vi "PROCEDURA TORSIOMETRO.vi"(6 "Text.Text":string="Prova QH: ", 7 "Tipo motore pompa":enum16{"Monofase", "Trifase"}(ring), 9 "Manuale F\\auto T":bool=TRUE, 10 "Status":refnum<vi>, 11 "input cluster":T1={"Scelta wattmetro"={"Wattmetro"=enum."No Selection"}, "SET RPM"=0.0, "SET TEMP"=0.0, "Array banchi"=[{"Nome"="Elettropompa", "Tors. scala1"=0, "Tors. scala2"=0, "rpm"=0, "TAMB"=0, "Indici Temperature"=[0, 1], "Indice freno"=1, "alimentatore trifase"=0, "alimentatore monofase"=0, "alimentatore dc arm"=0, "alimentatore dc ecc"=0, "alimentatore dc mp"=0}, {"Nome"="Sommersa", "Tors. scala1"=0, "Tors. scala2"=0, "rpm"=0, "TAMB"=1, "Indici Temperature"=[0, 1], "Indice freno"=0, "alimentatore trifase"=0, "alimentatore monofase"=0, "alimentatore dc arm"=0, "alimentatore dc ecc"=0, "alimentatore dc mp"=0}], "Array valvole linee avvio/fermata"=[], "banco selezionato"=0, "Nomi valvole prop sistema"=[], "canale-- sensore"=[], "Attriti B1"=[], "Attriti B2"=[], "Collegamento elettrico"={"ALIMENTAZIONE ELETTRICA"=enum."AC MONOFASE", "ID"=0, "#rami freddo\\eq term resmeter"=0, "#rami riscaldamento resmeter"=0, "#rami freddo\\eq term resistomat"=0, "#rami riscaldamento resistomat"=0, "CALCOLI"=enum."AC TRIFASE"}, "lingua"=0, "Costanti collaudo"={"P [bar]"=0.0, "T amb. [°C]"=0.0, "Umidità [%]"=0.0, "T acqua [°C] 2"=0.0}, "OPZIONI MISURE RES"={"MISURA A FREDDO"=enum."RESISTOMAT", "MISURA EQ. TERMICO"=enum."RESISTOMAT", "MISURA DT PROVA IN CORSO"=enum."RESISTOMAT - CON FERMATE", "MISURE PRIMA E DOPO"=enum."RESISTOMAT", "STRUMENTI PRESENTI"=enum."NESSUNO"}, "Dati targa motore"={"Vnom"=0.0, "Fnom"=0.0, "Inom"=0.0, "Cnom"=0.0, "Npoli"=0.0, "Scorta 1"=0.0, "Scorta 2"=0.0, "Scorta 3"=0.0}}) -> ()   [LabVIEW 2019]
uses:
  Global settings procedura tors.vi
  TypeDef/WT SELECTION.ctl
  TypeDef/Definizione linea.ctl
  TypeDef/Cluster INFO.ctl
  TypeDef/Collegamenti_elettrici.ctl
  TypeDef/Control Calcoli.ctl
panel:
  out "Fine":bool
  in  "Reset":bool
  in  "Stato auto":string
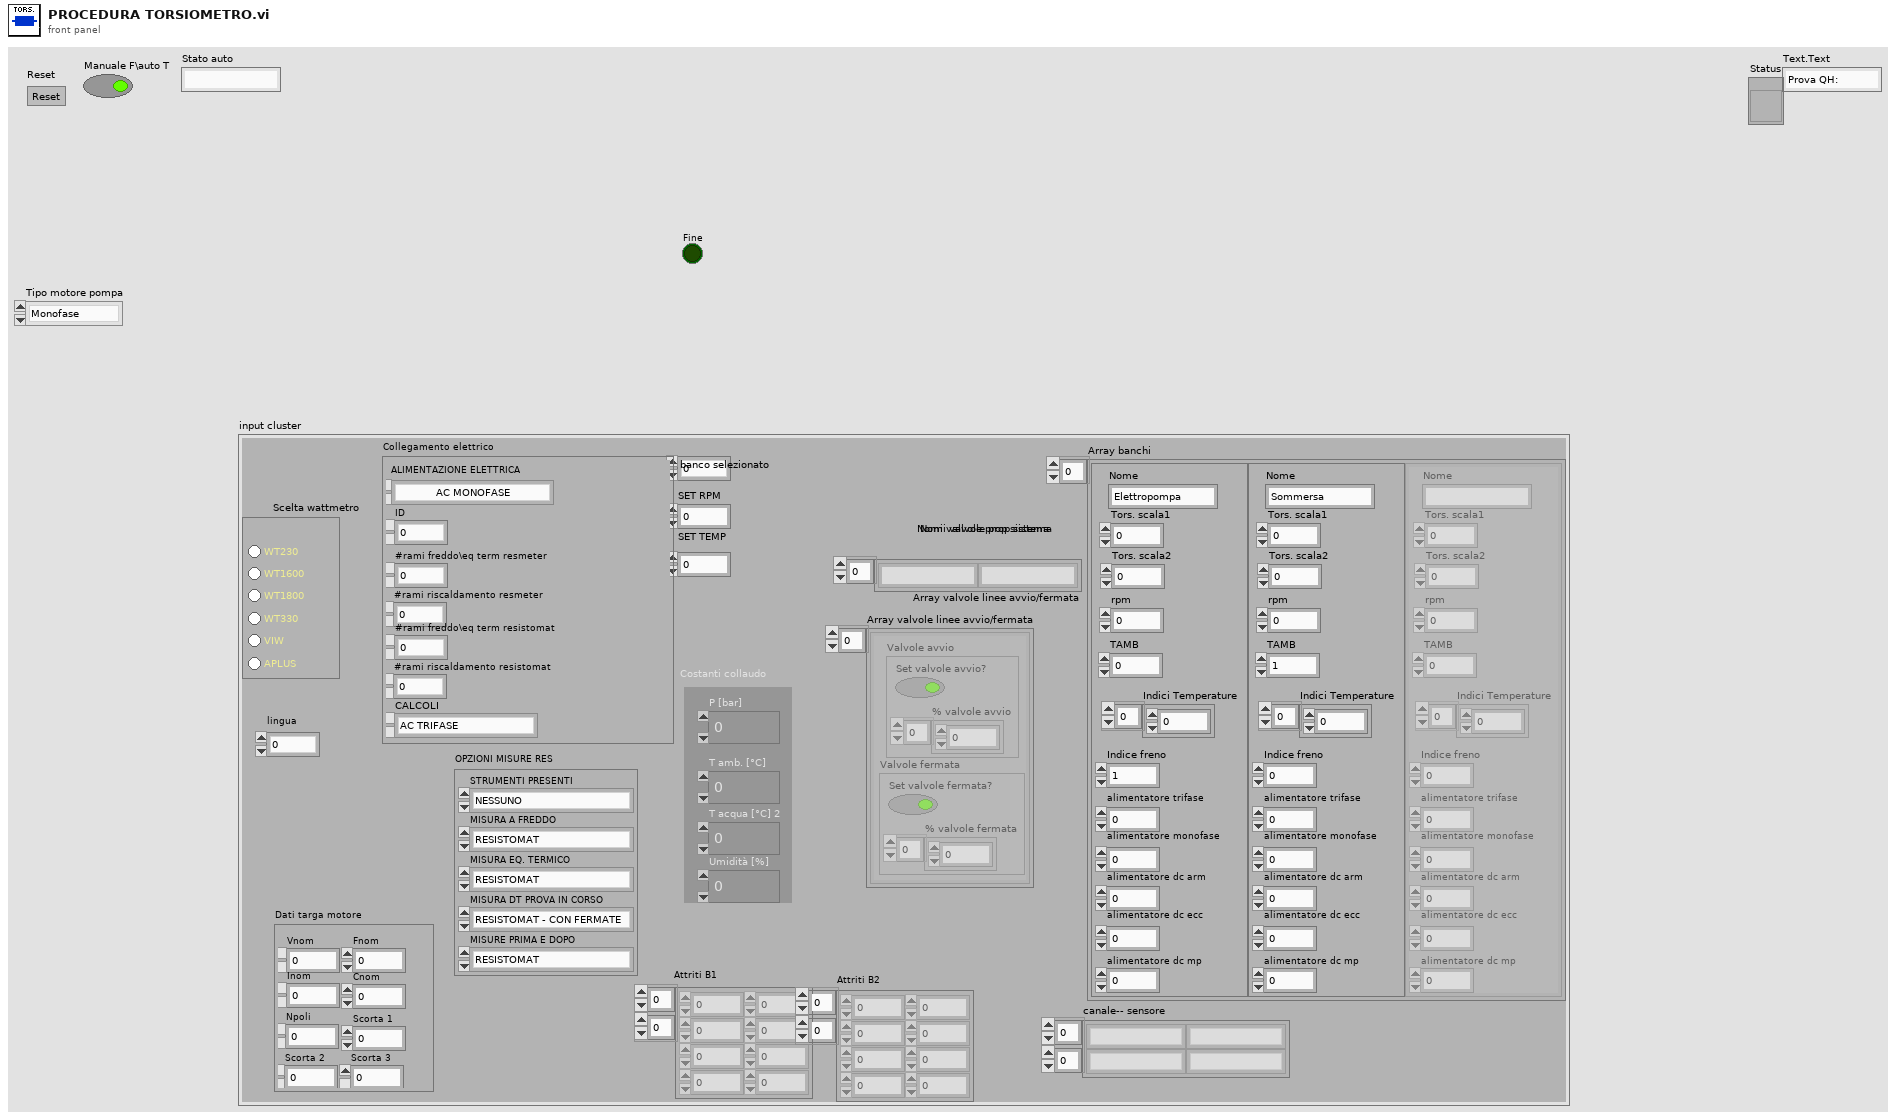
[diagram p1: front panel]
types:
  T1 = typedef "Cluster INFO.ctl" = cluster{"Scelta wattmetro":cluster{"Wattmetro":T2}, "SET RPM":dbl, "SET TEMP":dbl, "Array banchi":T3[], "Array valvole linee avvio/fermata":cluster{"Valvole avvio":cluster{"Set valvole avvio?":bool, "% valvole avvio":dbl[]}, "Valvole fermata":cluster{"Set valvole fermata?":bool, "% valvole fermata":dbl[]}}[], "banco selezionato":i8, "Nomi valvole prop sistema":string[], "canale-- sensore":string[][], "Attriti B1":dbl[][], "Attriti B2":dbl[][], "Collegamento elettrico":cluster{"ALIMENTAZIONE ELETTRICA":T4, "ID":i16, "#rami freddo\\eq term resmeter":i16, "#rami riscaldamento resmeter":i16, "#rami freddo\\eq term resistomat":i16, "#rami riscaldamento resistomat":i16, "CALCOLI":T5}, "lingua":i16, "Costanti collaudo":cluster{"P [bar]":dbl, "T amb. [°C]":dbl, "Umidità [%]":dbl, "T acqua [°C] 2":dbl}, "OPZIONI MISURE RES":cluster{"MISURA A FREDDO":enum16{"NESSUNO", "RESISTOMAT", "RES METER", "ENTRAMBI"}, "MISURA EQ. TERMICO":enum16{"NESSUNO", "RESISTOMAT", "RES METER", "ENTRAMBI"}, "MISURA DT PROVA IN CORSO":enum16{"NESSUNO", "RESISTOMAT - CON FERMATE", "RES METER - CON FERMATE", "RES METER - CONTINUO"}, "MISURE PRIMA E DOPO":enum16{"NESSUNO", "RESISTOMAT", "RES METER"}, "STRUMENTI PRESENTI":enum16{"NESSUNO", "RESISTOMAT", "RES METER", "ENTRAMBI"}}, "Dati targa motore":cluster{"Vnom":dbl, "Fnom":dbl, "Inom":dbl, "Cnom":dbl, "Npoli":dbl, "Scorta 1":dbl, "Scorta 2":dbl, "Scorta 3":dbl}}
  T2 = typedef "WT SELECTION.ctl" = enum32{"No Selection", "WT230", "WT1600", "WT1800", "WT330", "VIW", "APLUS"}
  T3 = typedef "Definizione linea.ctl" = cluster{"Nome":string, "Tors. scala1":i32, "Tors. scala2":i32, "rpm":i32, "TAMB":i32, "Indici Temperature":i16[], "Indice freno":i16, "alimentatore trifase":i16, "alimentatore monofase":i16, "alimentatore dc arm":i16, "alimentatore dc ecc":i16, "alimentatore dc mp":i16}
  T4 = typedef "Collegamenti_elettrici.ctl" = enum16{"AC TRIFASE", "AC TRIFASE + FRENO", "AC MONOFASE", "DC CON ECCITAZIONE", "DC CON ECCITAZIONE + FRENO", "DC NO ECCITAZIONE", "DC NO ECCITAZIONE + FRENO", "FRENO TRASC + AFE", "SOLO FRENO", "CARICO RESISTIVO", "GENERICO", "SOLO ACQUISITORE", "SCORTA 4", "SCORTA 5", "SCORTA 6"}
  T5 = typedef "Control Calcoli.ctl" = enum16{"AC TRIFASE", "AC MONOFASE", "DC ECCITAZIONE", "DC NO ECCITAZIONE", "POMPA TRIFASE", "POMPA MONOFASE", "GENERICO", "TRASFORMATORE", "ALTERNATORE TRASCINATO", "GRUPPO ELETTROGENO"}
  T6 = cluster{"Valvole avvio":cluster{"Set valvole avvio?":bool, "% valvole avvio":dbl[]}, "Valvole fermata":cluster{"Set valvole fermata?":bool, "% valvole fermata":dbl[]}}[]
  T7 = cluster{"rpm max":dbl, "Impostazioni procedura":cluster{"STEP RPM":dbl, "TEMPO DI\nSTABILIZZAZIONE [s]":dbl}}
  T8 = cluster{"Valvole avvio":cluster{"Set valvole avvio?":bool, "% valvole avvio":dbl[]}, "Valvole fermata":cluster{"Set valvole fermata?":bool, "% valvole fermata":dbl[]}}
  T9 = cluster{"Set valvole avvio?":bool, "% valvole avvio":dbl[]}
  T10 = cluster{"Set valvole fermata?":bool, "% valvole fermata":dbl[]}
  T11 = cluster{"Array of elements":cluster{"String":string, "variant":variant}[], "Single element":cluster{"String":string, "variant":variant}, "enque at\nopposite end (F)":bool, "no replications (F)":bool}
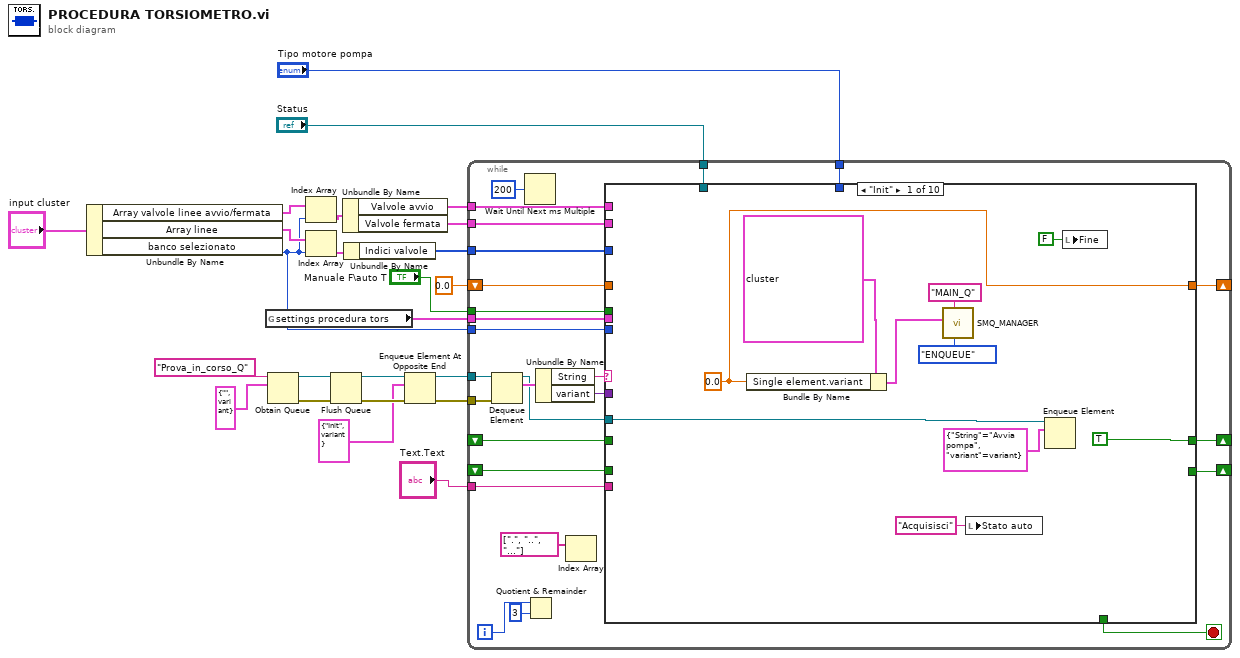
[diagram p0: block diagram]
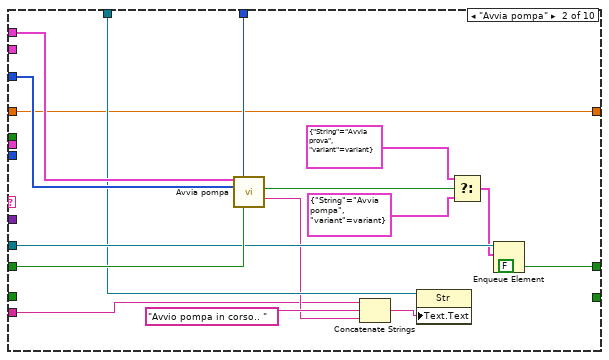
[diagram p2: hidden frame]
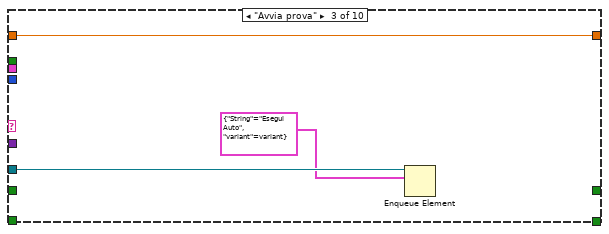
[diagram p3: hidden frame]
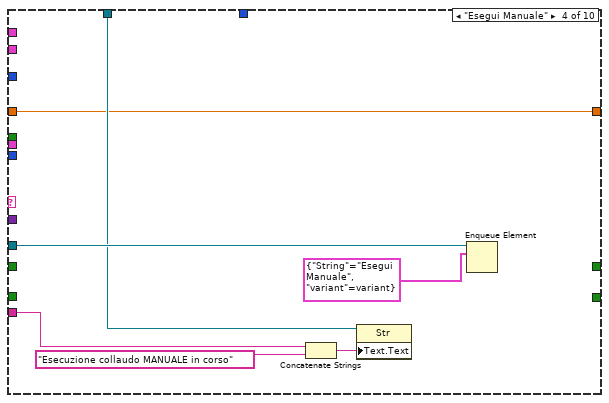
[diagram p4: hidden frame]
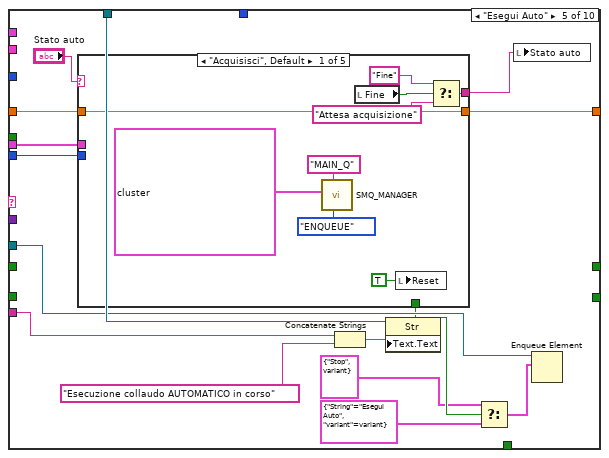
[diagram p5: hidden frame]
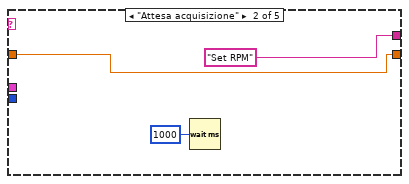
[diagram p6: hidden frame]
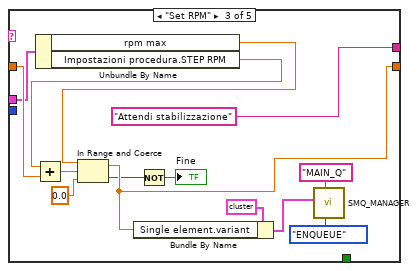
[diagram p7: hidden frame]
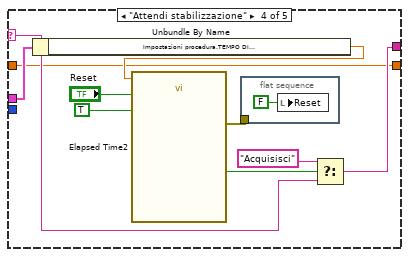
[diagram p8: hidden frame]
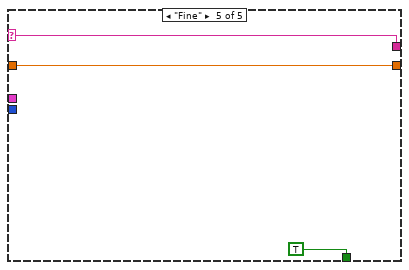
[diagram p9: hidden frame]
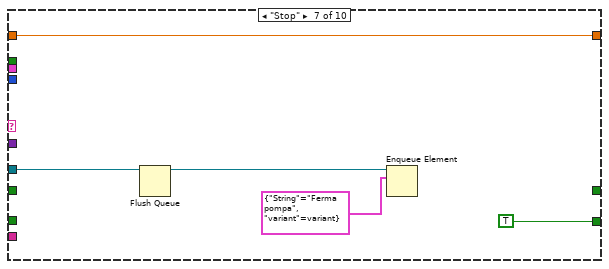
[diagram p11: hidden frame]
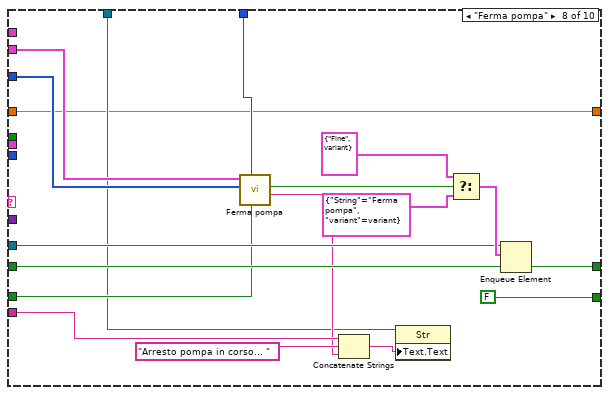
[diagram p12: hidden frame]
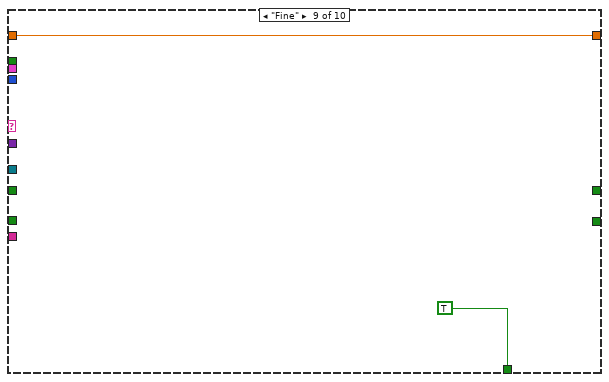
[diagram p13: hidden frame]
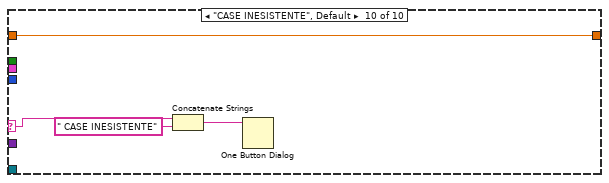
[diagram p14: hidden frame]
diagram:
  n1 = Unbundle By Name("input cluster") -> ("Array valvole linee avvio/fermata"=w11:T6, "Array linee"=w13:T3[], "banco selezionato"=w3:i8)
  n2 = global read "Global settings procedura tors.vi" "settings procedura tors"() -> (w2:T7)
  n3 = Obtain Queue(name (unnamed)="Prova_in_corso_Q" ("Queue Name"), element data type=cluster{"String":string, "variant":variant} {"String"="", "variant"=variant} ("element")) -> (queue out=w18:refnum<queue>, error out=w17:errorcluster)  [unwired: 3 in, 1 out]
  n4 = Index Array(array=w11, index=w3) -> (element=w10:T8)
  n5 = Index Array(array=w13, index=w3) -> (element=w12:T3)
  n6 = Flush Queue(queue=w18, error in (no error)=w17) -> (queue out=w22:refnum<queue>, error out=w21:errorcluster)  [unwired: 1 out]
  n7 = Unbundle By Name(w10) -> ("Valvole avvio"=w8:T9, "Valvole fermata"=w7:T10)
  n8 = Unbundle By Name(w12) -> ("Indici valvole"=w6:i16[])
  n9 = Enqueue Element At Opposite End(queue=w22, element=cluster{"String":string, "variant":variant} {"String"="Init", "variant"=variant}, error in (no error)=w21) -> (queue out=w24:refnum<queue>, error out=w23:errorcluster)  [unwired: 1 in, 1 out]
  n10 = while {
    tunnel: w24 -> [w50]
    tunnel: w23 -> [w49]
    tunnel: "Manuale F\\auto T" -> [w45]
    shift-right: [w43] -> _
    shift-left: _ -> [w42]
    tunnel: w8 -> [w41]
    tunnel: "Tipo motore pompa" -> [w40]
    tunnel: w7 -> [w39]
    shift-right: [w38] -> _
    shift-left: _ -> [w37]
    tunnel: w6 -> [w36]
    tunnel: "Status" -> [w35]
    tunnel: "Text.Text" -> [w33]
    tunnel: w3 -> [w28]
    tunnel: w2 -> [w27]
    shift-right: [w25] -> _
    shift-left: 0.0 -> [w26]
    i -> [w30]
    stop <- w34 stop-if-true
    n11 = Dequeue Element(queue=w50, error in (no error)=w49) -> (queue out=w44:refnum<queue>, element=w48:cluster{"String":string, "variant":variant})  [unwired: 1 in, 2 out]
    n12 = Wait Until Next ms Multiple(millisecond multiple=u32 200) -> ()  [unwired: 1 out]
    n13 = Quotient & Remainder(x=w30, y=3) -> ()  [unwired: 2 out]
    n14 = Unbundle By Name(w48) -> ("String"=w47:string, "variant"=w46:variant)
    n15 = Index Array(array=string[] [".", "..", "..."]) -> ()  [unwired: 1 in, 1 out]
    n16 = case shown="\"Init\"" w47 {
      selector: w47 -> [_ _ _ _ _ _ _ _ _ w170]
      tunnel: w46 -> [_ _ _ _ _ _ _ _ _ _]
      tunnel: w45 -> [_ _ _ _ _ _ _ _ _ _]
      tunnel: w44 -> [w60 w74 w79 w85 w95 _ w147 w157 _ _]
      tunnel: [TRUE FALSE _ _ _ _ _ w162 _ _] -> w43
      tunnel: w42 -> [_ w76 _ _ _ _ _ w162 _ _]
      tunnel: w41 -> [_ w68 _ _ _ _ _ _ _ _]
      tunnel: w40 -> [_ w69 _ _ _ _ _ w163 _ _]
      tunnel: w39 -> [_ _ _ _ _ _ _ w155 _ _]
      tunnel: [_ _ _ _ _ _ TRUE FALSE _ _] -> w38
      tunnel: w37 -> [_ _ _ _ _ _ _ w156 _ _]
      tunnel: w36 -> [_ w67 _ _ _ _ _ w154 _ _]
      tunnel: w35 -> [_ w66 _ w84 w99 _ _ w149 _ _]
      tunnel: [_ _ _ _ _ _ _ _ TRUE _] -> w34
      tunnel: w33 -> [_ w62 _ w83 w98 _ _ w152 _ _]
      tunnel: w28 -> [_ _ _ _ w90 _ _ _ _ _]
      tunnel: w27 -> [_ _ _ _ w89 _ _ _ _ _]
      tunnel: w26 -> [_ w61 w77 w80 w88 w142 w144 w148 w165 w167]
      tunnel: [w52 w61 w77 w80 w87 w142 w144 w148 w165 w167] -> w25
      frame "Init" {
        w52 = 0.0
        n17 = Bundle By Name(cluster=T11 {"Array of elements"=[], "Single element"={"String"="SET RPM INVERTER", "variant"=variant}, "enque at\nopposite end (F)"=FALSE, "no replications (F)"=FALSE} ("Enqueue cluster"), "Single element.variant"=w52) -> (w57:T11)
        n18 = call <userlib>:"SMQ_MANAGER.vi"("Function"=enum16{"INITIALIZE", "ENQUEUE", "STOP ALL"}."ENQUEUE", "Queue name"="MAIN_Q" ("Queue Name"), "Enqueue cluster"=w57) -> ()  [unwired: 8 in, 1 out]
        n19 = local write "Stato auto"("Acquisisci" ("Stato auto")) -> ()
        n20 = Enqueue Element(queue=w60, element=cluster{"String":string, "variant":variant} {"String"="Avvia pompa", "variant"=variant}) -> ()  [unwired: 2 in, 3 out]
        n21 = local write "Fine"(FALSE ("Fine")) -> ()
      }
      frame "Avvia pompa" {
        n22 = call "Avvia pompa.vi"("Valvole avvio"=w68, "Tipo motore pompa"=w69, "Indici valvole linea"=w67, "Reset avvio"=w76) -> ("Fine Avvio"=w73:bool, "stato"=w63:string)  [unwired: 10 in]
        n23 = Concatenate Strings(w62, "Avvio pompa in corso.. " ("Text.Text"), w63) -> (w64:string)
        n24 = property class="Str"(reference=w66, "Text.Text"=w64) -> ()  [unwired: 1 in, 2 out]
        n25 = Select(t=cluster{"String":string, "variant":variant} {"String"="Avvia prova", "variant"=variant} ("element"), s=w73, f=cluster{"String":string, "variant":variant} {"String"="Avvia pompa", "variant"=variant} ("element")) -> (s? t:f=w71:cluster{"String":string, "variant":variant})
        n26 = Enqueue Element(queue=w74, element=w71) -> ()  [unwired: 2 in, 3 out]
      }
      frame "Avvia prova" {
        n27 = Enqueue Element(queue=w79, element=cluster{"String":string, "variant":variant} {"String"="Esegui Auto", "variant"=variant}) -> ()  [unwired: 2 in, 3 out]
      }
      frame "Esegui Manuale" {
        n28 = Concatenate Strings(w83, "Esecuzione collaudo MANUALE in corso" ("string")) -> (w82:string)
        n29 = property class="Str"(reference=w84, "Text.Text"=w82) -> ()  [unwired: 1 in, 2 out]
        n30 = Enqueue Element(queue=w85, element=cluster{"String":string, "variant":variant} {"String"="Esegui Manuale", "variant"=variant}) -> ()  [unwired: 2 in, 3 out]
      }
      frame "Esegui Auto" {
        n31 = case shown="\"Acquisisci\", Default" "Stato auto" {
          selector: "Stato auto" -> [_ _ _ w133 w141]
          tunnel: [w106 "Set RPM" "Attendi stabilizzazione" w132 w141] -> w96
          tunnel: [_ _ _ _ TRUE] -> w92
          tunnel: w90 -> [_ _ _ _ _]
          tunnel: w89 -> [_ _ w122 w130 _]
          tunnel: w88 -> [w109 w111 w123 w128 w139]
          tunnel: [w109 w111 w117 w128 w139] -> w87
          frame "Acquisisci", Default {
            n32 = call <userlib>:"SMQ_MANAGER.vi"("Function"=enum16{"INITIALIZE", "ENQUEUE", "STOP ALL"}."ENQUEUE", "Queue name"="MAIN_Q" ("Queue Name"), "Enqueue cluster"=T11 {"Array of elements"=[], "Single element"={"String"="ACQUSIZIONE PROC TORS", "variant"=variant}, "enque at\nopposite end (F)"=FALSE, "no replications (F)"=FALSE}) -> ()  [unwired: 8 in, 1 out]
            n33 = local read "Fine"() -> (w108:bool)
            n34 = local write "Reset"(TRUE ("Reset")) -> ()
            n35 = Select(t="Fine", s=w108, f="Attesa acquisizione") -> (s? t:f=w106:string)
          }
          frame "Attesa acquisizione" {
            n36 = Wait (ms)(milliseconds to wait=u32 1000) -> ()  [unwired: 1 out]
          }
          frame "Set RPM" {
            n37 = Unbundle By Name(w122) -> ("rpm max"=w118:dbl, "Impostazioni procedura.STEP RPM"=w121:dbl)
            n38 = Add(x=w121, y=w123) -> (x+y=w120:dbl)
            n39 = In Range and Coerce(upper limit=w118, x=w120, lower limit=0.0) -> (coerced(x)=w117:dbl, In Range?=w116:bool)
            n40 = Bundle By Name(cluster=T11 {"Array of elements"=[], "Single element"={"String"="SET RPM INVERTER", "variant"=variant}, "enque at\nopposite end (F)"=FALSE, "no replications (F)"=FALSE} ("Enqueue cluster"), "Single element.variant"=w117) -> (w127:T11)
            n41 = Not(x=w116) -> (.not. x?=→"Fine":bool)
            n42 = call <userlib>:"SMQ_MANAGER.vi"("Function"=enum16{"INITIALIZE", "ENQUEUE", "STOP ALL"}."ENQUEUE", "Queue name"="MAIN_Q" ("Queue Name"), "Enqueue cluster"=w127) -> ()  [unwired: 8 in, 1 out]
          }
          frame "Attendi stabilizzazione" {
            n43 = Unbundle By Name(w130) -> ("Impostazioni procedura.TEMPO DI\nSTABILIZZAZIONE [s]"=w129:dbl)
            n44 = call "Elapsed Time2"("Time Target (s)"=w129, "Reset"="Reset", "Auto Reset"=TRUE) -> ("Time has Elapsed"=w134:bool, "error out"=w135:errorcluster)  [unwired: 9 in, 6 out]
            n45 = flat-sequence {
              tunnel: w135 -> [_]
              frame #0 {
                n46 = local write "Reset"(FALSE ("Reset")) -> ()
              }
            }
            n47 = Select(t="Acquisisci", s=w134, f=w133) -> (s? t:f=w132:string)
          }
          frame "Fine" {
          }
        }
        n48 = Concatenate Strings(w98, "Esecuzione collaudo AUTOMATICO in corso" ("string")) -> (w101:string)
        n49 = property class="Str"(reference=w99, "Text.Text"=w101) -> ()  [unwired: 1 in, 2 out]
        n50 = Select(t=cluster{"String":string, "variant":variant} {"String"="Stop", "variant"=variant} ("element"), s=w92, f=cluster{"String":string, "variant":variant} {"String"="Esegui Auto", "variant"=variant} ("element")) -> (s? t:f=w93:cluster{"String":string, "variant":variant})
        n51 = local write "Stato auto"(w96) -> ()
        n52 = Enqueue Element(queue=w95, element=w93) -> ()  [unwired: 2 in, 3 out]
      }
      frame "FINE ACQ" {
      }
      frame "Stop" {
        n53 = Flush Queue(queue=w147) -> (queue out=w146:refnum<queue>)  [unwired: 1 in, 2 out]
        n54 = Enqueue Element(queue=w146, element=cluster{"String":string, "variant":variant} {"String"="Ferma pompa", "variant"=variant}) -> ()  [unwired: 2 in, 3 out]
      }
      frame "Ferma pompa" {
        n55 = call "Ferma pompa.vi"("Reset fermata"=w156, "Tipo motore pompa"=w163, "Indici valvole linea"=w154, "Valvole fermata"=w155) -> ("stato"=w150:string, "Fine Fermata"=w158:bool)  [unwired: 6 in]
        n56 = Concatenate Strings(w152, "Arresto pompa in corso... " ("string"), w150) -> (w153:string)
        n57 = property class="Str"(reference=w149, "Text.Text"=w153) -> ()  [unwired: 1 in, 2 out]
        n58 = Select(t=cluster{"String":string, "variant":variant} {"String"="Fine", "variant"=variant} ("element"), s=w158, f=cluster{"String":string, "variant":variant} {"String"="Ferma pompa", "variant"=variant} ("element")) -> (s? t:f=w160:cluster{"String":string, "variant":variant})
        n59 = Enqueue Element(queue=w157, element=w160) -> ()  [unwired: 2 in, 3 out]
      }
      frame "Fine" {
      }
      frame "CASE INESISTENTE", Default {
        n60 = Concatenate Strings(w170, " CASE INESISTENTE" ("string")) -> (w169:string)
        n61 = One Button Dialog(message=w169) -> ()  [unwired: 1 in, 1 out]
      }
    }
  }
